vi "FPGA.vi"() -> ()   [LabVIEW 2018]
uses:
  PIC Select.ctl
  <vilib>/rvi/Emulation/niFpgaGetClockAttributes.vi
  <vilib>/rvi/Emulation/niFpgaSctlEmulationGetInTimedLoop.vi
  <vilib>/rvi/Emulation/niFpgaEmulationReportErrorSimple.vi
  <vilib>/rvi/eio/common/nirviEmuTemplateMethod_errors.vi
  <vilib>/rvi/Emulation/niFpgaCriticalErrorInLSC.vi
  <vilib>/eio/EIONode/EIONode.xnode
panel:
  in  "?":T1=enum."Voltage"
  in  "Pause":u8
  in  "Delay":u16
  in  "Write":bool
  out "PIC Monitor":u32
  in  "Data":u32
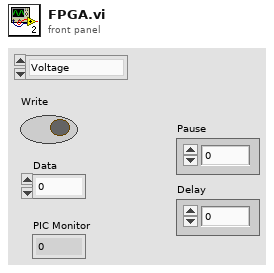
[diagram p1: front panel]
types:
  T1 = typedef "PIC Select.ctl" = enum16{"OFF", "Voltage", "Curtain", "Corona", "Heater"}
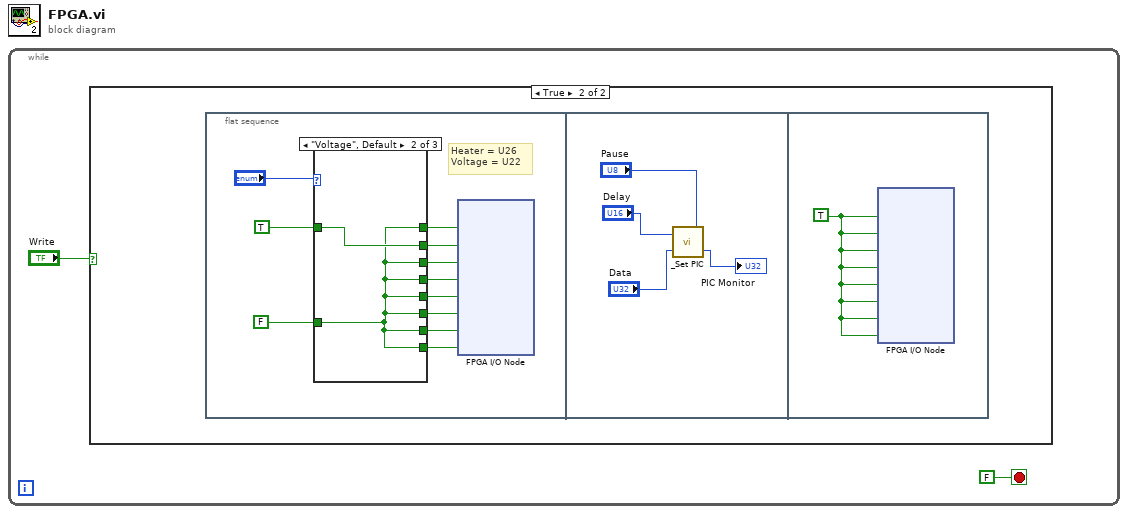
[diagram p0: block diagram]
diagram:
  n1 = while {
    stop <- FALSE stop-if-true
    n2 = case shown="True" "Write" {
      frame False {
      }
      frame True {
        n3 = flat-sequence {
          frame #0 {
            # "Heater = U26\nVoltage = U22"
            n4 = case shown="\"Voltage\", Default" "?" {
              tunnel: TRUE -> [w14 w16 w18]
              tunnel: FALSE -> [_ w15 w17]
              tunnel: [w14 w15 w18] -> w10
              tunnel: [w14 w15 w17] -> w9
              tunnel: [w14 w16 w17] -> w8
              tunnel: [w14 w15 w17] -> w7
              tunnel: [w14 w15 w17] -> w6
              tunnel: [w14 w15 w17] -> w5
              tunnel: [w14 w15 w17] -> w4
              tunnel: [w14 w15 w17] -> w3
              frame "OFF" {
              }
              frame "Voltage", Default {
              }
              frame "Heater" {
              }
            }
            n5 = xnode "FPGA I/O Node"("CS0"=w10, "CS1"=w8, "CS2"=w7, "BS0"=w6, "BS1"=w5, "BS2"=w4, "BS3"=w3, "BS4"=w9) -> ()  [unwired: 8 in, 8 out]
          }
          frame #1 {
            n6 = call "_Set PIC.vi"("Count(uSec)"="Pause", "Data"="Data", "Delay"="Delay") -> ("PIC Monitor"=→"PIC Monitor":u32)
          }
          frame #2 {
            w23 = TRUE
            n7 = xnode "FPGA I/O Node"("CS0"=w23, "CS1"=w23, "CS2"=w23, "BS0"=w23, "BS1"=w23, "BS2"=w23, "BS3"=w23, "BS4"=w23) -> ()  [unwired: 8 in, 8 out]
          }
        }
      }
    }
  }
